vi "Ex1_Add_COM.vi"() -> ()   [LabVIEW 2013]
panel:
  in  "Ex1_add.IClass1":refnum<k7>
  out "sum":dbl
  in  "b":dbl
  in  "a":dbl
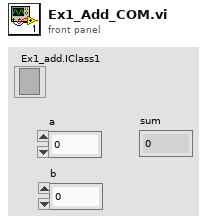
[diagram p1: front panel]
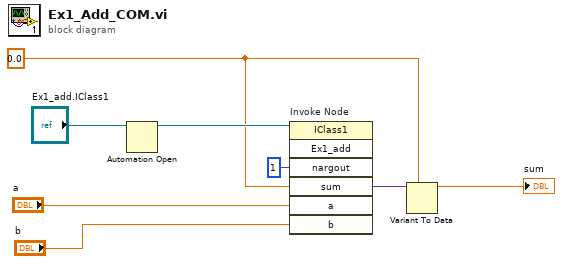
[diagram p0: block diagram]
diagram:
  w2 = 0.0
  n1 = Automation Open(Automation Refnum="Ex1_add.IClass1") -> (Automation Refnum=w8:refnum<k7>)  [unwired: 3 in, 1 out]
  n2 = invoke on="Invoke Node" class="IClass1" method="Ex1_add"(reference=w8, "nargout"=1, "sum"=w2, "a"="a", "b"="b") -> ("sum"=w7:variant)  [unwired: 2 in, 6 out]
  n3 = Variant To Data(type=w2, Variant=w7) -> (data=→"sum":dbl)  [unwired: 1 in, 1 out]
